vi "FPGA Phasor Measurement for M Class (50 Hz).vi"(0 "signal in":fxp<+/-,24,1>, 1 "number of channels":T3=1 items=["1"=1, "2"=2, "3"=3, "4"=4, "5"=5, "6"=6, "7"=7, "8"=8, "9"=9, "10"=10, "11"=11, "12"=12, "13"=13, "14"=14, "15"=15, "16"=16], 2 "memory information":T1, 5 "timestamp [s]":fxp<+,64,32> format="%#_42g", 7 "reference channel index (0)":u8, 9 "input valid? (T)":bool=TRUE, 12 "ready for output? (T)":bool=TRUE) -> (4 "output data":T2 {"timestamp [s]" format="%#.6g"; "phase [pi]" format="%#.6g"}, 10 "output valid?":bool, 14 "ready for input?":bool, 15 "error":i32)   [LabVIEW 2014, in "NI_EP_PMU_FPGA.lvlib"]
doc: "Calculates the instantaneous magnitude, phase, and frequency values of the fundamental frequency component as defined in the M class of performance in IEEE Std C37.118.1-2011. This VI resamples even-time-spaced voltage and current signals into even-angle-spaced signals. The input signals must have a sample rate of 50 kHz. The output rate is 24 samples per cycle. You must manually select the polymorphic instance to use."
uses:
  <vilib>/addons/Electrical Power/PMU/NI_EP_PMU_FPGA.lvlib
  <vilib>/addons/Electrical Power/PQ/Resampling/FPGA/subVIs/fpga_NofCH.ctl
  <vilib>/addons/Electrical Power/PQ/Resampling/NI_EP_Resample_FPGA.lvlib
  <vilib>/addons/Electrical Power/PMU/FPGA/subVIs/fpga_OutputDataType.ctl
  <vilib>/addons/Electrical Power/PMU/FPGA/subVIs/fpga_Memory Information (M Class_50Hz).ctl
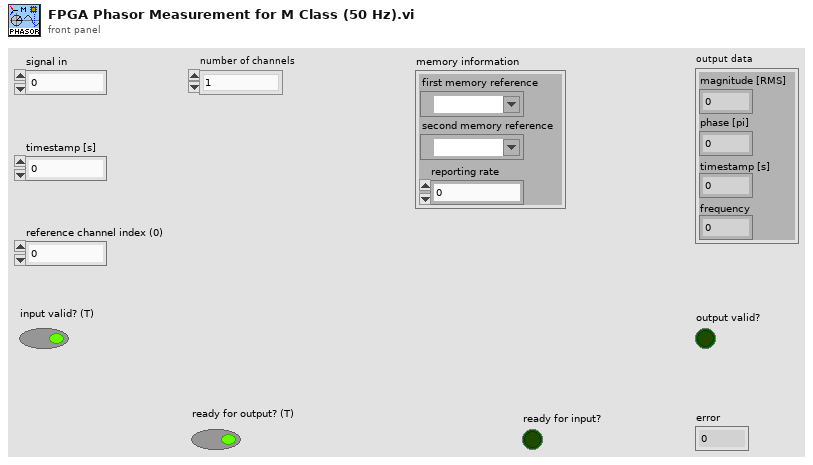
[diagram p1: front panel]
types:
  T1 = typedef "NI_EP_PMU_FPGA.lvlib/fpga_Memory Information (M Class_50Hz).ctl" = cluster{"first memory reference":refnum<k21>, "second memory reference":refnum<k21>, "reporting rate":i16}
  T2 = typedef "NI_EP_PMU_FPGA.lvlib/fpga_OutputDataType.ctl" = cluster{"magnitude [RMS]":fxp<+,32,6>, "phase [pi]":fxp<+/-,32,2>, "timestamp [s]":fxp<+,64,32>, "frequency":fxp<+,32,8>}
  T3 = typedef "NI_EP_Resample_FPGA.lvlib/fpga_NofCH.ctl" = u8
  T4 = typedef "NI_EP_Resample_FPGA.lvlib/fpga_Resampled.ctl" = cluster{"signal":fxp<+/-,32,3>, "timestamp [s]":fxp<+,64,32>, "frequency":fxp<+,32,8>}
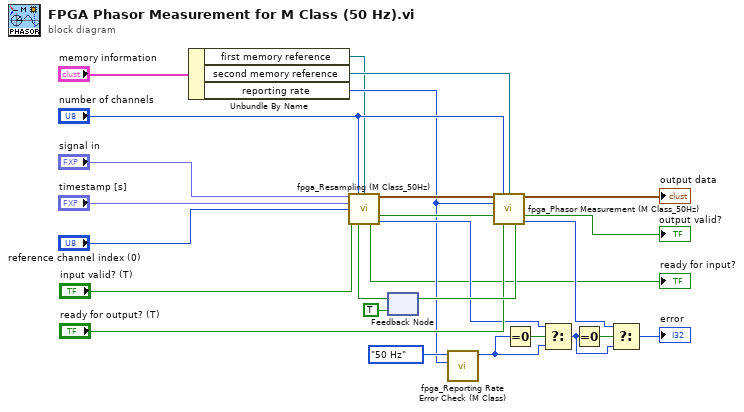
[diagram p0: block diagram]
diagram:
  n1 = Unbundle By Name("memory information") -> ("first memory reference"=w1:refnum<k21>, "second memory reference"=w12:refnum<k21>, "reporting rate"=w8:i16)
  n2 = feedback #1(TRUE ("ready for input")) -> (w18:bool)
  n3 = call <vilib>:"fpga_Resampling (M Class_50Hz).vi"("signal in"="signal in", "number of channels"="number of channels", "Memory In"=w1, "timestamp [s]"="timestamp [s]", "reference channel index"="reference channel index (0)", "input data valid? (T)"="input valid? (T)", "ready for output? (T)"=w18) -> ("resampled data"=w23:T4, "output valid"=w22:bool, "ready for input"=→"ready for input?":bool, "error"=w10:i32)  [unwired: 5 in]
  n4 = call <vilib>:"fpga_Reporting Rate Error Check (M Class).vi"("reporting rate"=w8, "nominal frequency"=enum16{"50 Hz", "60 Hz"}."50 Hz") -> ("error"=w9:i32)  [unwired: 9 in]
  n5 = call <vilib>:"fpga_Phasor Measurement (M Class_50Hz).vi"("resampled data"=w23, "number of channels"="number of channels", "Memory In"=w12, "reporting rate"=w8, "input valid? (T)"=w22, "ready for output? (T)"="ready for output? (T)") -> ("output data"=→"output data":T2, "output valid"=→"output valid?":bool, "ready for input"=w20:bool, "error"=w6:i32)  [unwired: 6 in]
  n6 = feedback-in #1(w20) -> ()
  n7 = Equal To 0?(x=w9) -> (x = 0?=w11:bool)
  n8 = Select(t=w10, s=w11, f=w9) -> (s? t:f=w5:i32)
  n9 = Equal To 0?(x=w5) -> (x = 0?=w7:bool)
  n10 = Select(t=w6, s=w7, f=w5) -> (s? t:f=→"error":i32)
